vi "Connect.vi"(8 "error in (no error)":errorcluster, 11 "Hitronics in":refnum<class "Hitronics.lvclass">) -> (0 "error out":errorcluster, 3 "Hitronics out":refnum<class "Hitronics.lvclass">)   [LabVIEW 2018, in "Hitronics.lvlib" / "Hitronics.lvclass"]
doc: "Connect to Laser over specified VISA Resource"
uses:
  Hitronics.lvclass
  Program Files/National Instruments/LabVIEW 2018/examples/Instrument IO/Serial/support/Serial - Settings.ctl
  <vilib>/Instr/_visa.llb/VISA Configure Serial Port (Instr).vi
  PPLs/Laser/Parent/Laser.lvlibp/Laser.lvclass
  C:/AME Test Engineering/LabVIEW/PPLs/Laser/Parent/Laser.lvlibp/Laser.lvclass
panel:
  in  "Serial Settings":T1={"baud rate"=115200, "data bits"=8, "parity"=enum."None", "stop bits"=10, "flow control"=0} {"flow control" items=["None"=0, "XON/XOFF"=1, "RTS/CTS"=2, "DTR/DSR"=4]; "stop bits" items=["1.0"=10, "1.5"=15, "2.0"=20]; "data bits" min=5 max=8 step=1; "baud rate" items=["75"=75, "110"=110, "134"=134, "150"=150, "300"=300, "600"=600, "1200"=1200, "1800"=1800, "2400"=2400, "4800"=4800, "7200"=7200, "9600"=9600, "14400"=14400, "19200"=19200, "28800"=28800, "38400"=38400, "56000"=56000, "57600"=57600, "115200"=115200, "128000"=128000, "230400"=230400]}
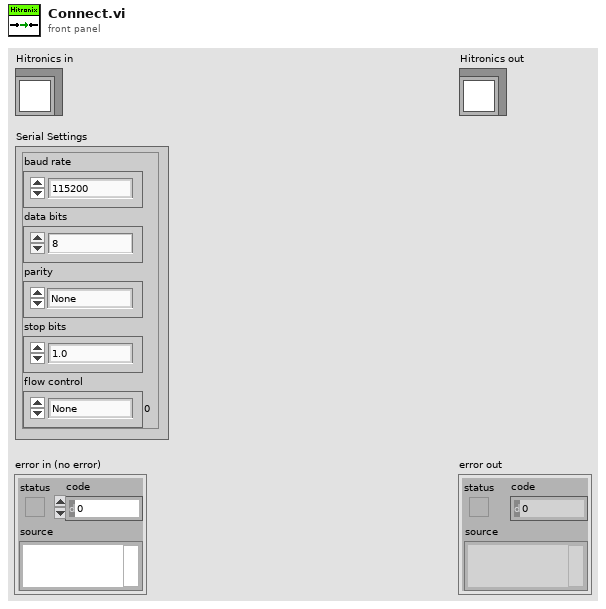
[diagram p1: front panel]
types:
  T1 = typedef "Hitronics.lvlib/Hitronics.lvclass/Serial - Settings.ctl" = cluster{"baud rate":u32, "data bits":u16, "parity":enum16{"None", "Odd", "Even", "Mark", "Space"}, "stop bits":u16, "flow control":u16}
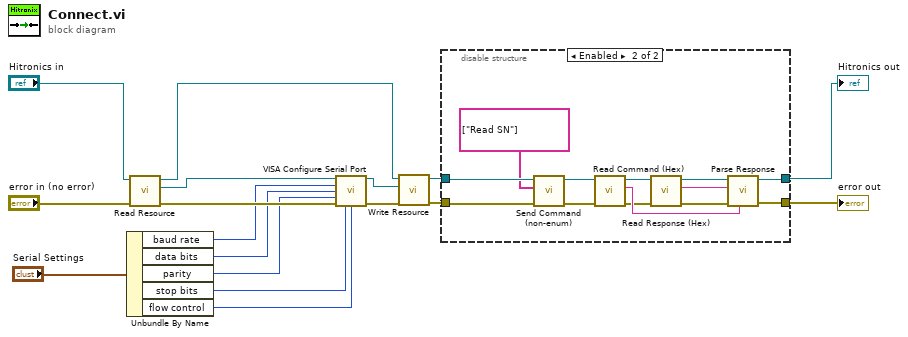
[diagram p0: block diagram]
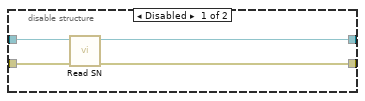
[diagram p2: hidden frame]
diagram:
  n1 = Unbundle By Name("Serial Settings") -> ("baud rate"=w13:u32, "data bits"=w12:u16, "parity"=w11:enum16{"None", "Odd", "Even", "Mark", "Space"}, "stop bits"=w10:u16, "flow control"=w9:u16)
  n2 = call "Read Resource.vi"("error in (no error)"="error in (no error)", "Laser in"="Hitronics in") -> ("error out"=w14:errorcluster, "Resource"=w15:refnum<visa-resource-name>, "Laser out"=w6:refnum<class "Hitronics.lvclass">)  [unwired: 7 in]
  n3 = call-poly "VISA Configure Serial Port"("VISA resource name"=w15, "baud rate (9600)"=w13, "data bits (8)"=w12, "parity (0:none)"=w11, "error in (no error)"=w14, "stop bits (10: 1 bit)"=w10, "flow control (0:none)"=w9) -> ("VISA resource name out"=w8:refnum<visa-resource-name>, "error out"=w5:errorcluster)  [unwired: 2 in, 5 out]
  n4 = call "Write Resource.vi"("error in (no error)"=w5, "Resource"=w8, "Laser in"=w6) -> ("error out"=w4:errorcluster, "Laser out"=w3:refnum<class "Hitronics.lvclass">)  [unwired: 7 in]
  n5 = disable-structure shown="Enabled" {
    disable-tunnel: w4 -> [w21 w33]
    disable-tunnel: w3 -> [w20 w34]
    disable-tunnel: [w19 w24] -> w2
    disable-tunnel: [w18 w23] -> w1
    frame Disabled {
      n6 = call "Read SN.vi"("error in (no error)"=w21, "Hitronics in"=w20) -> ("error out"=w18:errorcluster, "Hitronics out"=w19:refnum<class "Hitronics.lvclass">)  [unwired: 8 in]
    }
    frame Enabled {
      n7 = call-dynamic "Send Command (non-enum).vi"("error in (no error)"=w33, "Commands"=string[] ["Read SN"], "Hitronics in"=w34) -> ("error out"=w26:errorcluster, "Hitronics out"=w30:refnum<class "Hitronics.lvclass">)  [unwired: 7 in]
      n8 = call-dynamic "Read Command (Hex).vi"("error in (no error)"=w26, "Hitronics in"=w30) -> ("error out"=w27:errorcluster, "Command (Hex)"=w29:string, "Hitronics out"=w28:refnum<class "Hitronics.lvclass">)  [unwired: 7 in]
      n9 = call-dynamic "Read Response (Hex).vi"("error in (no error)"=w27, "Hitronics in"=w28) -> ("error out"=w22:errorcluster, "Response (Hex)"=w31:string, "Hitronics out"=w25:refnum<class "Hitronics.lvclass">)  [unwired: 7 in]
      n10 = call "Parse Response.vi"("Command String (Hex)"=w29, "error in (no error)"=w22, "Response String (Hex)"=w31, "Hitronics in"=w25) -> ("error out"=w23:errorcluster, "Hitronics out"=w24:refnum<class "Hitronics.lvclass">)  [unwired: 5 in, 1 out]
    }
  }
  "error out" <- w1
  "Hitronics out" <- w2
